vi "Send Message.vi"(6 "priority":i32, 8 "error in (no error)":errorcluster, 9 "timeout ms (-1)":i32=-1, 10 "Message":refnum<class "Message.lvclass">, 11 "Error Stream in":refnum<class "Error Stream.lvclass">) -> (0 "error out":errorcluster, 3 "Error Stream out":refnum<class "Error Stream.lvclass">)   [LabVIEW 2020, in "Error Stream.lvclass"]
doc: "Override this method to specify the action the local copy of this object will perform to send a message to its remote counterpart."
uses:
  Error Stream.lvclass
  <vilib>/ActorFramework/Message/Message.lvclass
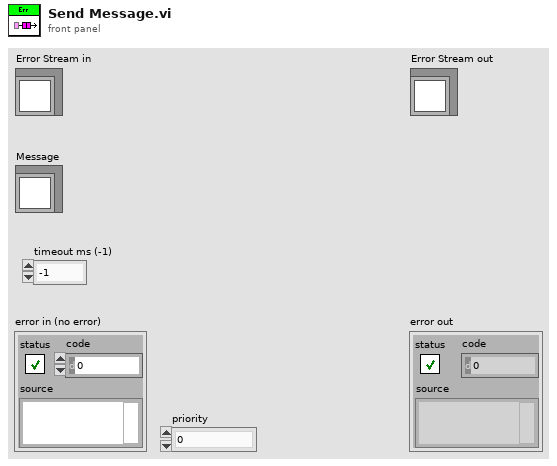
[diagram p1: front panel]
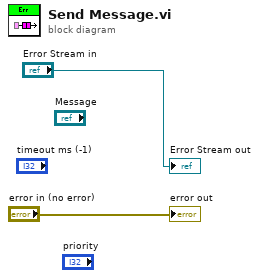
[diagram p0: block diagram]
diagram:
  "error out" <- "error in (no error)"
  "Error Stream out" <- "Error Stream in"
